vi "MetaClientQueue.vi"() -> ()   [LabVIEW 2017]
uses:
  QueueControl.ctl
panel:
  in  "QueueRef":refnum<vi>
  in  "QueueChanged":bool=TRUE
  in  "QueueControl":T1
  # "Queue :"
  # "Queue :"
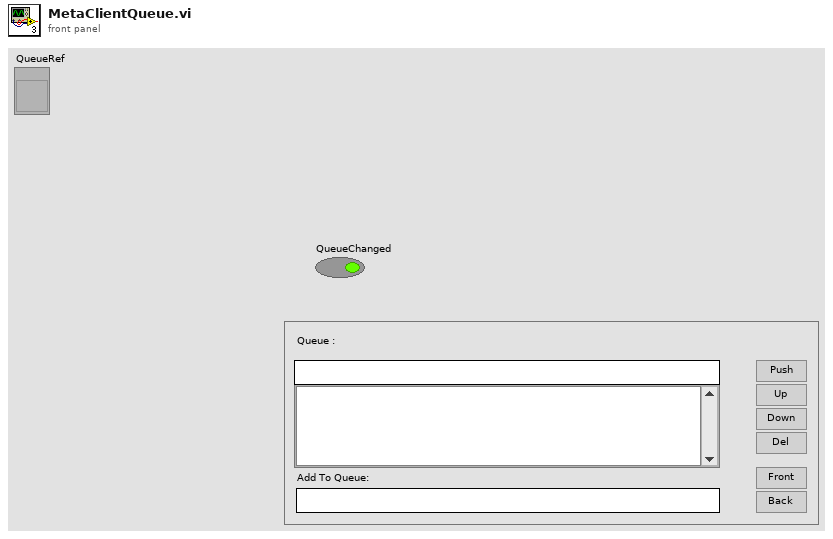
[diagram p1: front panel]
types:
  T1 = typedef "QueueControl.ctl" = cluster{"QueueFromServer":i32, "First Queue":string, "Add To Queue:":string, "Up":bool, "Down":bool, "Del":bool, "Front":bool, "Back":bool, "Next":bool}
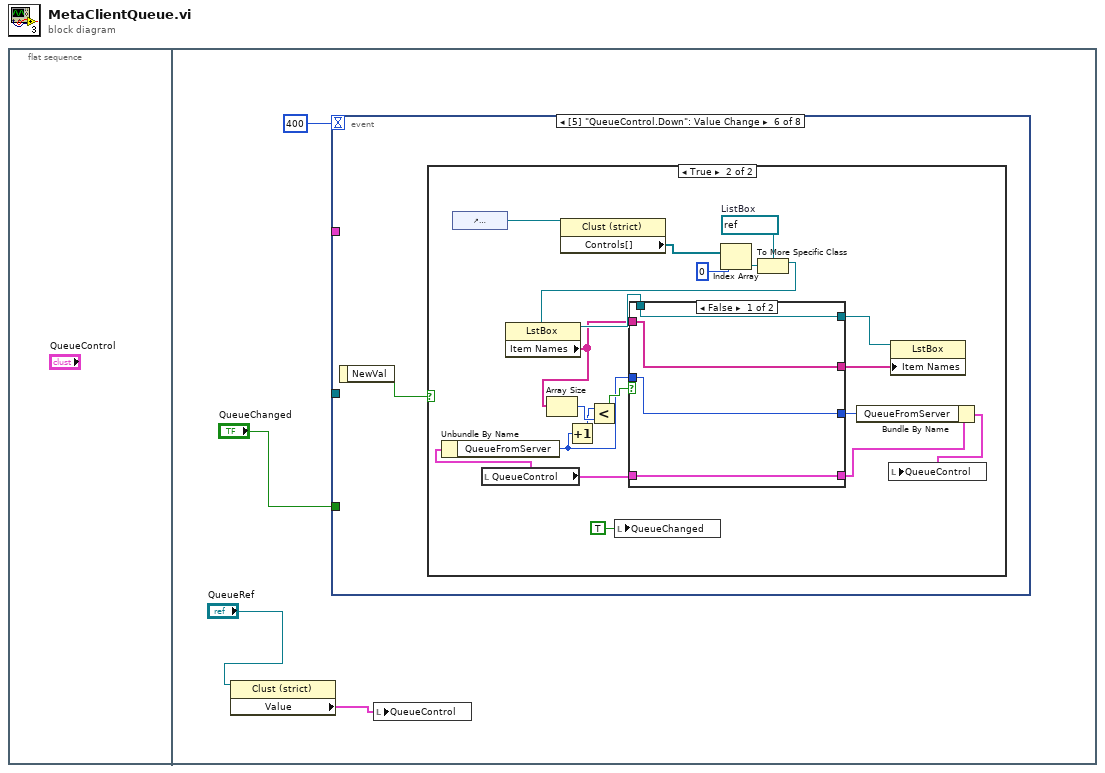
[diagram p0: block diagram]
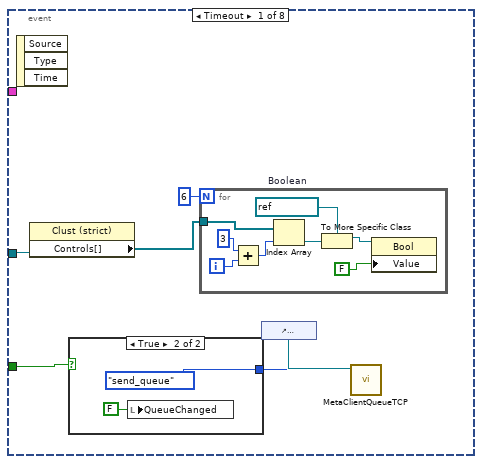
[diagram p2: hidden frame]
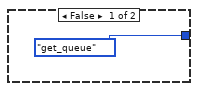
[diagram p3: hidden frame]
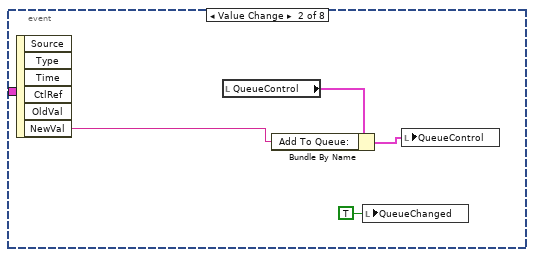
[diagram p4: hidden frame]
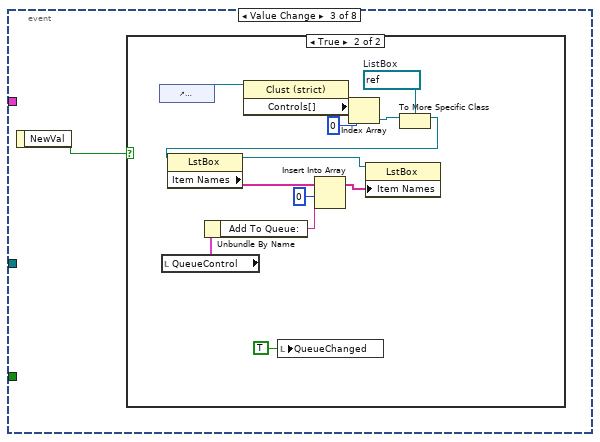
[diagram p5: hidden frame]
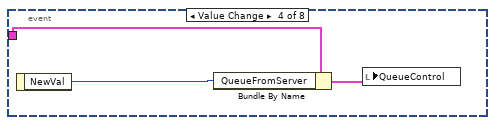
[diagram p7: hidden frame]
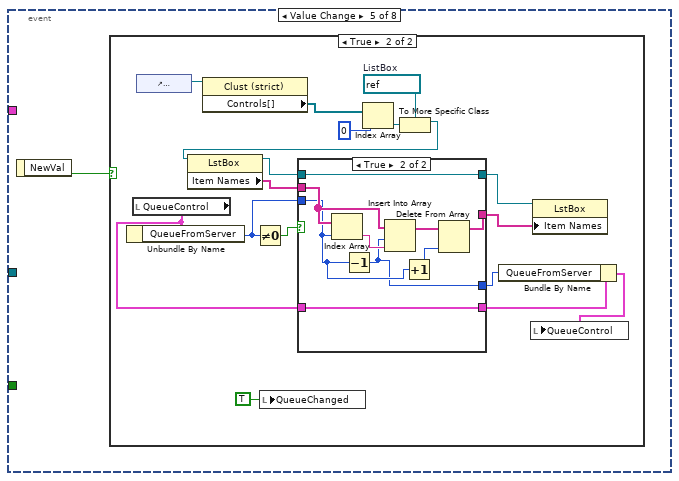
[diagram p8: hidden frame]
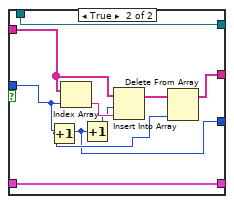
[diagram p12: hidden frame]
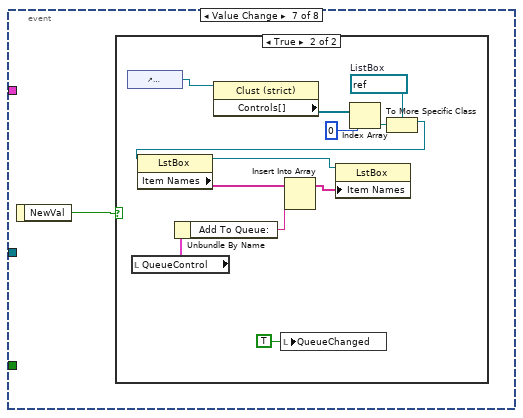
[diagram p13: hidden frame]
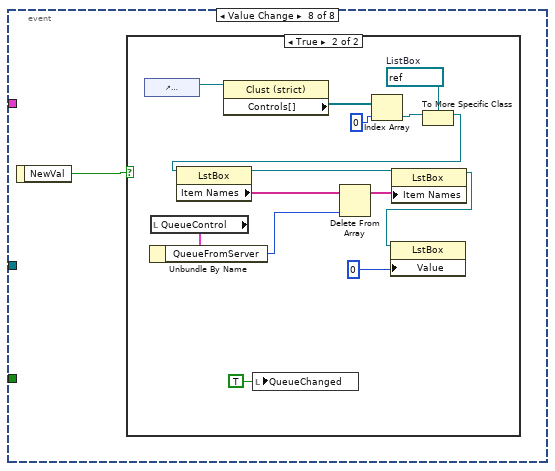
[diagram p15: hidden frame]
diagram:
  n1 = flat-sequence {
    frame #0 {
    }
    frame #1 {
      n2 = property class="Clust (strict)"(reference="QueueRef") -> ("Value"=w2:T1)  [unwired: 1 in, 2 out]
      n3 = event shown="[5] \"QueueControl.Down\": Value Change" {
        selector: _ -> [_ _ _ _ _ _ _ _]
        dyn-events: _ -> [_ _ _ _ _ _ _ _]
        timeout: 400 -> [_ _ _ _ _ _ _ _]
        tunnel: _ -> [w11 _ _ w43 _ _ _ _]
        tunnel: "QueueChanged" -> [w8 _ _ _ _ _ _ _]
        tunnel: _ -> [w7 _ _ _ _ _ _ _]
        event Timeout {
          n4 = event-data() -> ()  [unwired: 1 in, 3 out]
          n5 = property class="Clust (strict)"(reference=w7) -> ("Controls[]"=w5:refnum<vi>[])  [unwired: 1 in, 2 out]
          n6 = case shown="True" w8 {
            tunnel: [enum16{"shutdown", "send_queue", "get_queue"}."get_queue" ("Enum") enum16{"shutdown", "send_queue", "get_queue"}."send_queue" ("Enum")] -> w9
            frame False {
            }
            frame True {
              n7 = local write "QueueChanged"(FALSE ("QueueChanged")) -> ()
            }
          }
          n8 = for {
            N: 6 -> [_]
            tunnel: w5 -> [w16]
            i -> [w19]
            w13 = refnum<vi> refnum  # Boolean
            n9 = Add(x=3, y=w19) -> (x+y=w17:i32)
            n10 = Index Array(array=w16, index=w17) -> (element=w15:refnum<vi>)
            n11 = To More Specific Class(target class=w13, reference=w15) -> (specific class reference=w14:refnum<vi>)  [unwired: 1 in, 1 out]
            n12 = property class="Bool"(reference=w14, "Value"=FALSE) -> ()  [unwired: 1 in, 2 out]
          }
          n13 = control-ref of="QueueControl"() -> (w10:refnum<vi>)
          n14 = call "MetaClientQueueTCP.vi"("Enum"=w9, "RefIn"=w10) -> ()  [unwired: 8 in, 2 out]
        }
        event Value Change {
          n15 = event-data() -> ("NewVal"=w26:string)  [unwired: 1 in, 5 out]
          n16 = local read "QueueControl"() -> (w25:T1)
          n17 = Bundle By Name(cluster=w25, "Add To Queue:"=w26) -> (w24:T1)
          n18 = local write "QueueChanged"(TRUE ("QueueChanged")) -> ()
          n19 = local write "QueueControl"(w24) -> ()
        }
        event Value Change {
          n20 = event-data() -> ("NewVal"=w27:bool)  [unwired: 1 in]
          n21 = case shown="True" w27 {
            frame False {
            }
            frame True {
              w35 = refnum<vi> refnum  # ListBox
              n22 = control-ref of="QueueControl"() -> (w40:refnum<vi>)
              n23 = local read "QueueControl"() -> (w33:T1)
              n24 = Unbundle By Name(w33) -> ("Add To Queue:"=w32:string)
              n25 = property on="Property Node" class="Clust (strict)"(reference=w40) -> ("Controls[]"=w39:refnum<vi>[])  [unwired: 1 in, 2 out]
              n26 = local write "QueueChanged"(TRUE ("QueueChanged")) -> ()
              n27 = Index Array(array=w39, index=0) -> (element=w37:refnum<vi>)
              n28 = To More Specific Class(target class=w35, reference=w37) -> (specific class reference=w36:refnum<vi>)  [unwired: 1 in, 1 out]
              n29 = property on="Property Node" class="LstBox"(reference=w36) -> (reference out=w31:refnum<vi>, "Item Names"=w34:string[])  [unwired: 1 in, 1 out]
              n30 = Insert Into Array(array=w34, index=0, new element=w32) -> (w30:string[])
              n31 = property on="Property Node" class="LstBox"(reference=w31, "Item Names"=w30) -> ()  [unwired: 1 in, 2 out]
            }
          }
        }
        event Value Change {
          n32 = event-data() -> ("NewVal"=w42:i32)  [unwired: 1 in]
          n33 = Bundle By Name(cluster=w43, "QueueFromServer"=w42) -> (w41:cluster{})
          n34 = local write "QueueControl"(w41) -> ()
        }
        event Value Change {
          n35 = event-data() -> ("NewVal"=w44:bool)  [unwired: 1 in]
          n36 = case shown="True" w44 {
            frame False {
            }
            frame True {
              w58 = refnum<vi> refnum  # ListBox
              n37 = local read "QueueControl"() -> (w49:T1)
              n38 = Unbundle By Name(w49) -> ("QueueFromServer"=w53:i32)
              n39 = control-ref of="QueueControl"() -> (w61:refnum<vi>)
              n40 = property class="Clust (strict)"(reference=w61) -> ("Controls[]"=w57:refnum<vi>[])  [unwired: 1 in, 2 out]
              n41 = Not Equal To 0?(x=w53) -> (x != 0?=w55:bool)
              n42 = local write "QueueChanged"(TRUE ("QueueChanged")) -> ()
              n43 = Index Array(array=w57, index=0) -> (element=w59:refnum<vi>)
              n44 = To More Specific Class(target class=w58, reference=w59) -> (specific class reference=w56:refnum<vi>)  [unwired: 1 in, 1 out]
              n45 = property on="Property Node" class="LstBox"(reference=w56) -> (reference out=w51:refnum<vi>, "Item Names"=w54:string[])  [unwired: 1 in, 1 out]
              n46 = case shown="True" w55 {
                tunnel: w54 -> [w65 w74]
                tunnel: w53 -> [w62 w69]
                tunnel: [w65 w71] -> w52
                tunnel: w51 -> [w64 w68]
                tunnel: [w64 w68] -> w50
                tunnel: w49 -> [w63 w67]
                tunnel: [w63 w67] -> w48
                tunnel: [w62 w66] -> w47
                frame False {
                }
                frame True {
                  n47 = Index Array(array=w74, index=w69) -> (element=w73:string)
                  n48 = Decrement(x=w69) -> (x-1=w66:i32)
                  n49 = Insert Into Array(array=w74, index=w66, new element=w73) -> (w72:string[])
                  n50 = Increment(x=w69) -> (x+1=w70:i32)
                  n51 = Delete From Array(array=w72, index=w70) -> (array with subset deleted=w71:string[])  [unwired: 1 in, 1 out]
                }
              }
              n52 = Bundle By Name(cluster=w48, "QueueFromServer"=w47) -> (w46:T1)
              n53 = local write "QueueControl"(w46) -> ()
              n54 = property on="Property Node" class="LstBox"(reference=w50, "Item Names"=w52) -> ()  [unwired: 1 in, 2 out]
            }
          }
        }
        event Value Change {
          n55 = event-data() -> ("NewVal"=w75:bool)  [unwired: 1 in]
          n56 = case shown="True" w75 {
            frame False {
            }
            frame True {
              w92 = refnum<vi> refnum  # ListBox
              n57 = control-ref of="QueueControl"() -> (w90:refnum<vi>)
              n58 = local read "QueueControl"() -> (w86:T1)
              n59 = Unbundle By Name(w86) -> ("QueueFromServer"=w77:i32)
              n60 = property class="Clust (strict)"(reference=w90) -> ("Controls[]"=w91:refnum<vi>[])  [unwired: 1 in, 2 out]
              n61 = Increment(x=w77) -> (x+1=w78:i32)
              n62 = local write "QueueChanged"(TRUE ("QueueChanged")) -> ()
              n63 = Index Array(array=w91, index=0) -> (element=w93:refnum<vi>)
              n64 = To More Specific Class(target class=w92, reference=w93) -> (specific class reference=w89:refnum<vi>)  [unwired: 1 in, 1 out]
              n65 = property on="Property Node" class="LstBox"(reference=w89) -> (reference out=w82:refnum<vi>, "Item Names"=w80:string[])  [unwired: 1 in, 1 out]
              n66 = Array Size(array=w80) -> (size(s)=w79:i32)
              n67 = Less?(x=w78, y=w79) -> (x < y?=w88:bool)
              n68 = case shown="False" w88 {
                tunnel: w77 -> [w96 w100]
                tunnel: w80 -> [w97 w105]
                tunnel: [w96 w99] -> w87
                tunnel: w86 -> [w95 w104]
                tunnel: [w95 w104] -> w85
                tunnel: [w97 w103] -> w83
                tunnel: w82 -> [w98 w102]
                tunnel: [w98 w102] -> w81
                frame False {
                }
                frame True {
                  n69 = Increment(x=w100) -> (x+1=w99:i32)
                  n70 = Index Array(array=w105, index=w100) -> (element=w107:string)
                  n71 = Increment(x=w99) -> (x+1=w101:i32)
                  n72 = Insert Into Array(array=w105, index=w101, new element=w107) -> (w106:string[])
                  n73 = Delete From Array(array=w106, index=w100) -> (array with subset deleted=w103:string[])  [unwired: 1 in, 1 out]
                }
              }
              n74 = Bundle By Name(cluster=w85, "QueueFromServer"=w87) -> (w84:T1)
              n75 = local write "QueueControl"(w84) -> ()
              n76 = property on="Property Node" class="LstBox"(reference=w81, "Item Names"=w83) -> ()  [unwired: 1 in, 2 out]
            }
          }
        }
        event Value Change {
          n77 = event-data() -> ("NewVal"=w108:bool)  [unwired: 1 in]
          n78 = case shown="True" w108 {
            frame False {
            }
            frame True {
              w117 = refnum<vi> refnum  # ListBox
              n79 = control-ref of="QueueControl"() -> (w111:refnum<vi>)
              n80 = local read "QueueControl"() -> (w115:T1)
              n81 = Unbundle By Name(w115) -> ("Add To Queue:"=w114:string)
              n82 = property on="Property Node" class="Clust (strict)"(reference=w111) -> ("Controls[]"=w120:refnum<vi>[])  [unwired: 1 in, 2 out]
              n83 = local write "QueueChanged"(TRUE ("QueueChanged")) -> ()
              n84 = Index Array(array=w120, index=0) -> (element=w118:refnum<vi>)
              n85 = To More Specific Class(target class=w117, reference=w118) -> (specific class reference=w110:refnum<vi>)  [unwired: 1 in, 1 out]
              n86 = property on="Property Node" class="LstBox"(reference=w110) -> (reference out=w113:refnum<vi>, "Item Names"=w116:string[])  [unwired: 1 in, 1 out]
              n87 = Insert Into Array(array=w116, new element=w114) -> (w112:string[])  [unwired: 1 in]
              n88 = property on="Property Node" class="LstBox"(reference=w113, "Item Names"=w112) -> ()  [unwired: 1 in, 2 out]
            }
          }
        }
        event Value Change {
          n89 = event-data() -> ("NewVal"=w121:bool)  [unwired: 1 in]
          n90 = case shown="True" w121 {
            frame False {
            }
            frame True {
              w133 = refnum<vi> refnum  # ListBox
              n91 = control-ref of="QueueControl"() -> (w135:refnum<vi>)
              n92 = local read "QueueControl"() -> (w128:T1)
              n93 = Unbundle By Name(w128) -> ("QueueFromServer"=w127:i32)
              n94 = property class="Clust (strict)"(reference=w135) -> ("Controls[]"=w132:refnum<vi>[])  [unwired: 1 in, 2 out]
              n95 = local write "QueueChanged"(TRUE ("QueueChanged")) -> ()
              n96 = Index Array(array=w132, index=0) -> (element=w134:refnum<vi>)
              n97 = To More Specific Class(target class=w133, reference=w134) -> (specific class reference=w130:refnum<vi>)  [unwired: 1 in, 1 out]
              n98 = property class="LstBox"(reference=w130) -> (reference out=w125:refnum<vi>, "Item Names"=w129:string[])  [unwired: 1 in, 1 out]
              n99 = Delete From Array(array=w129, index=w127) -> (array with subset deleted=w126:string[])  [unwired: 1 in, 1 out]
              n100 = property class="LstBox"(reference=w125, "Item Names"=w126) -> (reference out=w124:refnum<vi>)  [unwired: 1 in, 1 out]
              n101 = property class="LstBox"(reference=w124, "Value"=0) -> ()  [unwired: 1 in, 2 out]
            }
          }
        }
      }
      n102 = local write "QueueControl"(w2) -> ()
    }
  }
